vi "WPI_AnalogChannelOpen.vi"(8 "error in (no error)":errorcluster, 10 "Analog Channel":T1=enum."AI 1") -> (0 "error out":errorcluster, 3 "AIDeviceRef":T2={"DevStatus"={"status"=FALSE, "code"=0, "source"=""}, "Analog Channel"=enum."Invalid"})   [LabVIEW 2017]
doc: "Opens a reference to the analog channel you specify. You must open a reference before using any other AnalogChannel VIs.\n\nThis software is licensed. Open the labview\\readme\\WPI Robotics Library Open Source License.txt file for more information."
uses:
  <vilib>/Rock Robotics/WPI/AnalogChannel/WPI_AnalogChannelDevRef.ctl
  <vilib>/Rock Robotics/SystemInterfaces/AI/FPGA_AIChannel.ctl
  <vilib>/Rock Robotics/WPI/AnalogChannel/WPI_AnalogChannelChannelCacheOp.ctl
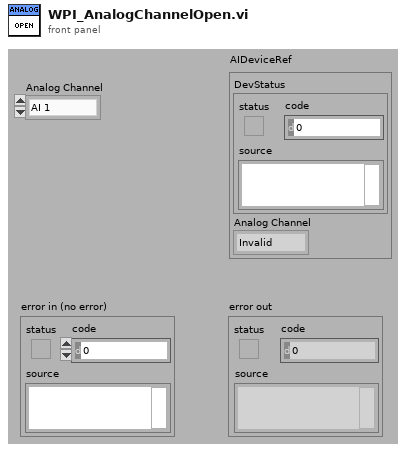
[diagram p1: front panel]
types:
  T1 = typedef "FPGA_AIChannel.ctl" = enum8{"AI 0", "AI 1", "AI 2", "AI 3", "AI MXP 0", "AI MXP 1", "AI MXP 2", "AI MXP 3", "Invalid"}
  T2 = typedef "WPI_AnalogChannelDevRef.ctl" = cluster{"DevStatus":errorcluster, "Analog Channel":T1}
  T3 = typedef "WPI_AnalogChannelChannelCacheOp.ctl" = enum16{"Acquire", "Release", "Status"}
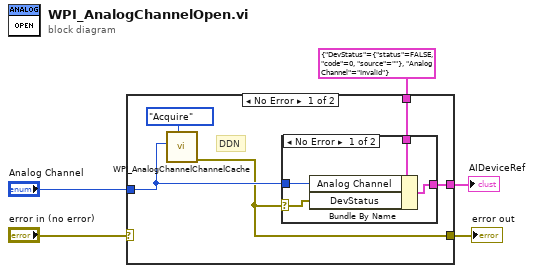
[diagram p0: block diagram]
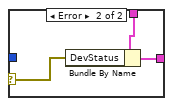
[diagram p2: hidden frame]
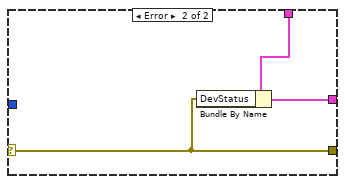
[diagram p3: hidden frame]
diagram:
  n1 = case shown="No Error" "error in (no error)" {
    selector: "error in (no error)" -> [_ w18]
    tunnel: T2 {"DevStatus"={"status"=FALSE, "code"=0, "source"=""}, "Analog Channel"=enum."Invalid"} ("AIDeviceRef") -> [w10 w20]
    tunnel: [w9 w19] -> w4
    tunnel: "Analog Channel" -> [w8 _]
    tunnel: [w6 w18] -> w1
    frame No Error {
      # "DDN"
      n2 = call <vilib>:"WPI_AnalogChannelChannelCache.vi"("Operation"=WPI_AnalogChannelChannelCacheOp."Acquire", "Channel"=w8) -> ("error out"=w6:errorcluster)  [unwired: 2 in, 7 out]
      n3 = case shown="No Error" w6 {
        selector: w6 -> [w11 w15]
        tunnel: w10 -> [w14 w17]
        tunnel: [w13 w16] -> w9
        tunnel: w8 -> [w12 _]
        frame No Error {
          n4 = Bundle By Name(cluster=w14, "Analog Channel"=w12, "DevStatus"=w11) -> (w13:T2)
        }
        frame Error {
          n5 = Bundle By Name(cluster=w17, "DevStatus"=w15) -> (w16:T2)
        }
      }
    }
    frame Error {
      n6 = Bundle By Name(cluster=w20, "DevStatus"=w18) -> (w19:T2)
    }
  }
  "AIDeviceRef" <- w4
  "error out" <- w1
